vi "Ejercicio3_Hipotenusa.vi"() -> ()   [LabVIEW 2022 SP3]
panel:
  in  "stop":bool
  out "Hipotenusa":dbl
  in  "Cateto Adyacente":dbl
  in  "Cateto Opuesto":dbl
  # "Hipotenusa"
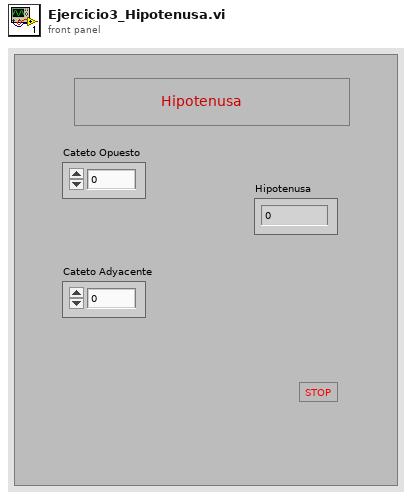
[diagram p1: front panel]
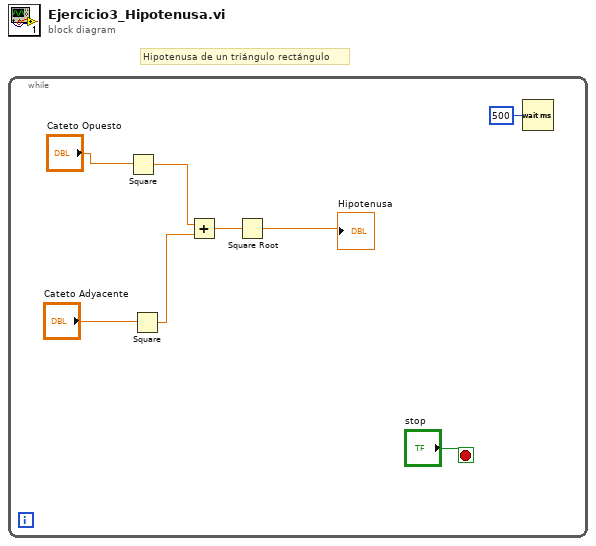
[diagram p0: block diagram]
diagram:
  # "Hipotenusa de un triángulo rectángulo"
  n1 = while {
    stop <- "stop" stop-if-true
    n2 = Square(x="Cateto Opuesto") -> (x^2=w5:dbl)
    n3 = Square(x="Cateto Adyacente") -> (x^2=w4:dbl)
    n4 = Add(x=w5, y=w4) -> (x+y=w3:dbl)
    n5 = Square Root(x=w3) -> (sqrt(x)=→"Hipotenusa":dbl)
    n6 = Wait (ms)(milliseconds to wait=u32 500) -> ()  [unwired: 1 out]
  }
